vi "DaqDigital_ConfigurationLines.vi"(8 "error in":errorcluster, 10 "Canales":tag[](array[tag]), 11 "DAQ Board Name":tag) -> (0 "error out":errorcluster, 3 "task out":refnum<k21>)   [LabVIEW 2020]
uses:
  <vilib>/DAQmx/create/channels.llb/DAQmx Create Channel (DI-Digital Input).vi
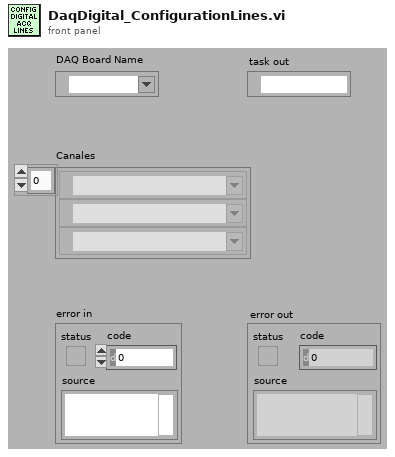
[diagram p1: front panel]
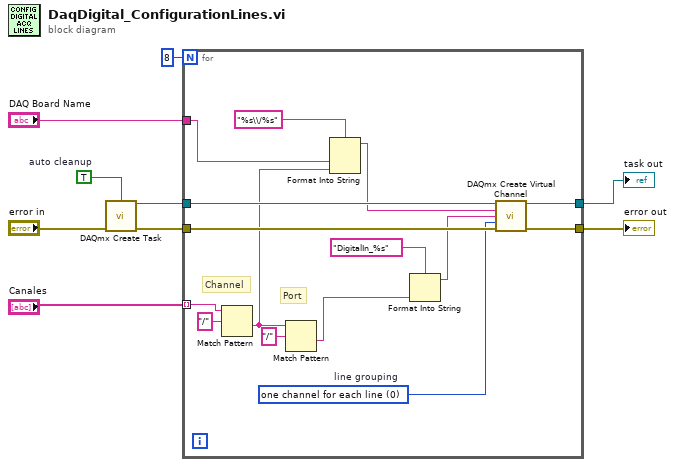
[diagram p0: block diagram]
diagram:
  w7 = TRUE  # auto cleanup
  n1 = call <vilib>:"DAQmx Create Task.vi"("auto cleanup"=w7, "error in"="error in") -> ("task out"=w6:refnum<k21>, "error out"=w8:errorcluster)  [unwired: 12 in]
  n2 = for {
    N: 8 -> [_]
    tunnel: w8 -> [w24]
    tunnel: w6 -> [w23]
    tunnel: "DAQ Board Name" -> [w19]
    tunnel: "Canales" -> [w13] mode=indexing
    tunnel: [w12] -> w2
    tunnel: [w11] -> w3
    w22 = 0 items=["one channel for each line", "one channel for all lines"]  # line grouping
    # "Port"
    # "Channel"
    n3 = Match Pattern(string=w13, regular expression="/") -> (after substring=w10:string)  [unwired: 1 in, 3 out]
    n4 = Match Pattern(string=w10, regular expression="/") -> (after substring=w15:string)  [unwired: 1 in, 3 out]
    n5 = Format Into String(format string="%s\\/%s", w19, w10) -> (resulting string=w18:string)  [unwired: 2 in, 1 out]
    n6 = Format Into String(format string="DigitalIn_%s", w15) -> (resulting string=w14:string)  [unwired: 2 in, 1 out]
    n7 = call-poly <vilib>:"DAQmx Create Virtual Channel.vi"("task in"=w23, "lines"=w18, "name to assign"=w14, "line grouping"=w22, "error in"=w24) -> ("task out"=w12:refnum<k21>, "error out"=w11:errorcluster)  [unwired: 9 in]
  }
  "error out" <- w3
  "task out" <- w2
